vi "Open Serial Session.vi"(7 "Mode (RTU)":enum16{"RTU", "ASCII"}(ring), 8 "Error in":errorcluster caption="Error in (no error)", 9 "Slave ID":u8=1, 10 "Serial Config":T1={"baud rate (bps)"=19200, "stop bits"=10, "parity"=0, "flow control"=0, "timeout"=1000, "retries"=1} {"stop bits" items=["1.0"=10, "1.5"=15, "2.0"=20]; "flow control" items=["None", "XON/XOFF", "RTS/CTS", "XON/XOFF & RTS/CTS", "DTR/DSR", "XON/XOFF & DTR/DSR"]; "parity" items=["None", "Odd", "Even", "Mark", "Space"]}, 11 "VISA Resource":refnum<visa-resource-name>) -> (0 "Error out":errorcluster, 3 "MB_Serial session":refnum<class "MB_Master_Serial.lvclass">)   [LabVIEW 2016, in "MB Master.lvlib" / "MB_Master_Serial.lvclass"]
doc: "Opens a new modbus session and initializes the serial port. Note that the slave ID can be changed later via the property node \"Slave ID\"."
uses:
  MB_Master_Serial.lvclass
  MB_Master_Serial.lvclass/MB_Master_Serial.ctl
  MB_ADU/MB_ADU.lvclass/MB_ADU.ctl
  MB_ADU_RTU/MB_ADU_RTU.lvclass/MB_ADU_RTU.ctl
  MB_ADU/Build ADU.vi
  MB_ADU_RTU/MB_ADU_RTU.lvclass
  C:/Users/PRANAV/Downloads/Modbus-Master-master (7)/Modbus-Master-master/MB_ADU/MB_ADU.lvclass
  C:/Users/PRANAV/Downloads/Modbus-Master-master (7)/Modbus-Master-master/MB_ADU_Serial/MB_ADU_Serial.lvclass
  MB_VISA_Lock/MB_VISA_Lock.lvlib
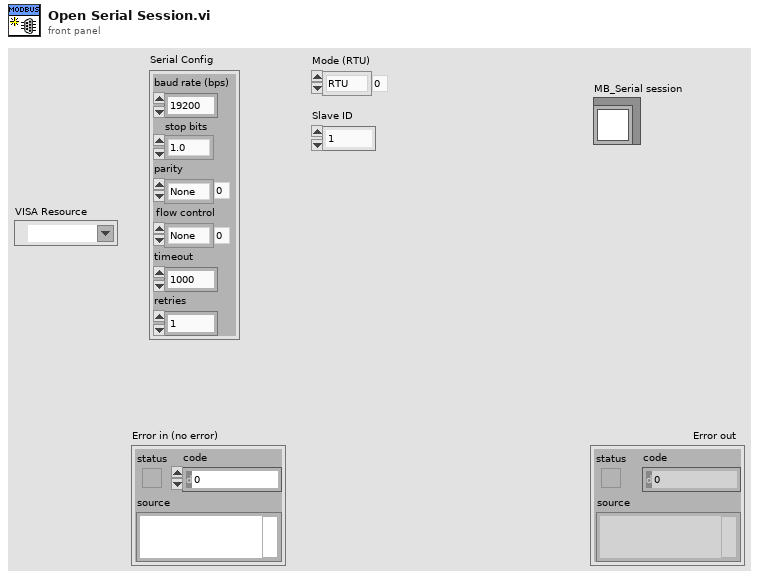
[diagram p1: front panel]
types:
  T1 = cluster{"baud rate (bps)":u32, "stop bits":u16, "parity":u16, "flow control":u16, "timeout":u32, "retries":i32}
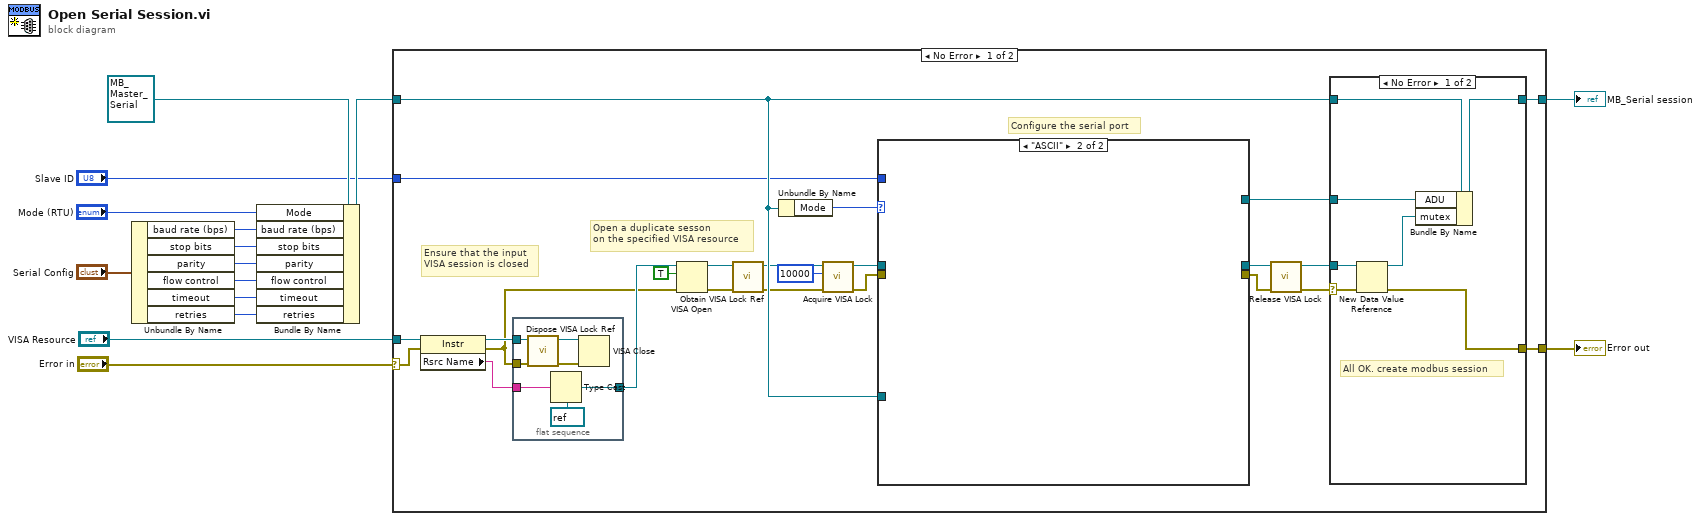
[diagram p0: block diagram]
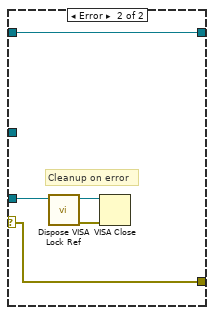
[diagram p2: hidden frame]
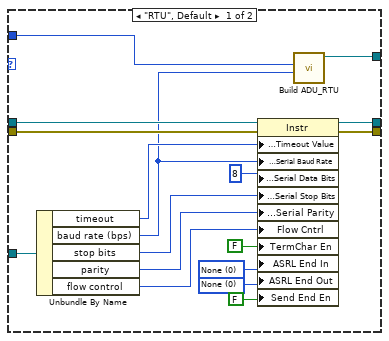
[diagram p3: hidden frame]
diagram:
  n1 = Unbundle By Name("Serial Config") -> ("baud rate (bps)"=w13:u32, "stop bits"=w12:u16, "parity"=w11:u16, "flow control"=w10:u16, "timeout"=w9:u32, "retries"=w8:i32)
  n2 = Bundle By Name(cluster=refnum<class "MB_Master_Serial.lvclass"> refnum ("MB_Serial session"), "Mode"="Mode (RTU)", "baud rate (bps)"=w13, "stop bits"=w12, "parity"=w11, "flow control"=w10, "timeout"=w9, "retries"=w8) -> (w6:refnum<class "MB_Master_Serial.lvclass">)
  n3 = case shown="No Error" "Error in" {
    selector: "Error in" -> [w31 w76]
    tunnel: [w39 w77] -> w5
    tunnel: w6 -> [w37 w77]
    tunnel: [w33 w76] -> w4
    tunnel: "Slave ID" -> [w34 _]
    tunnel: "VISA Resource" -> [w32 _]
    frame No Error {
      # "Configure the serial port"
      # "Open a duplicate sesson\non the specified VISA resource"
      # "Ensure that the input \nVISA session is closed"
      n4 = property class="Instr"(reference=w32, error in=w31) -> (reference out=w21:refnum<visa-resource-name>, error out=w18:errorcluster, "Rsrc Name"=w20:string)
      n5 = flat-sequence {
        tunnel: w21 -> [w57]
        tunnel: w18 -> [w56]
        tunnel: w20 -> [w53]
        tunnel: [w52] -> w19
        frame #0 {
          n6 = call "Dispose VISA Lock Ref.vi"("error in (no error)"=w56, "VISA session in"=w57) -> ("error out"=w55:errorcluster, "VISA session out"=w58:refnum<visa-resource-name>)  [unwired: 8 in]
          n7 = Type Cast(type=refnum<visa-resource-name> refnum ("VISA Resource"), x=w53) -> (*(type *) &x=w52:refnum<visa-resource-name>)
          n8 = VISA Close(VISA resource name=w58, error in (no error)=w55) -> ()  [unwired: 1 out]
        }
      }
      n9 = VISA Open(duplicate session (F)=TRUE, error in (no error)=w18, VISA resource name=w19) -> (VISA resource name=w30:refnum<visa-resource-name>, error out=w29:errorcluster)  [unwired: 2 in]
      n10 = call "Obtain VISA Lock Ref.vi"("error in (no error)"=w29, "VISA session in"=w30) -> ("error out"=w28:errorcluster, "VISA session out"=w27:refnum<visa-resource-name>)  [unwired: 8 in]
      n11 = Unbundle By Name(w37) -> ("Mode"=w36:enum16{"RTU", "ASCII"})
      n12 = call "Acquire VISA Lock.vi"("error in (no error)"=w28, "timeout in ms (-1)"=10000, "VISA resource name"=w27) -> ("error out"=w24:errorcluster, "VISA resource name out"=w26:refnum<visa-resource-name>)  [unwired: 7 in]
      n13 = case shown="\"ASCII\"" w36 {
        tunnel: [w61 _] -> w38
        tunnel: w26 -> [w75 _]
        tunnel: w24 -> [w74 _]
        tunnel: w37 -> [w73 _]
        tunnel: [w68 _] -> w23
        tunnel: [w63 _] -> w22
        tunnel: w34 -> [w59 _]
        frame "RTU", Default {
          w64 = u16 0 items=["None", "Last Bit", "TermChar", "Break"] ("Serial Settings:End Mode for Writes")
          w65 = u16 0 items=["None", "Last Bit", "TermChar"] ("Serial Settings:End Mode for Reads")
          n14 = Unbundle By Name(w73) -> ("timeout"=w72:u32, "baud rate (bps)"=w60:u32, "stop bits"=w71:u16, "parity"=w70:u16, "flow control"=w69:u16)
          n15 = property class="Instr"(reference=w75, error in=w74, "General Settings:Timeout Value"=w72, "Serial Settings:Serial Baud Rate"=w60, "Serial Settings:Serial Data Bits"=u16 8 ("Serial Settings:Data Bits"), "Serial Settings:Serial Stop Bits"=w71, "Serial Settings:Serial Parity"=w70, "Flow Cntrl"=w69, "TermChar En"=FALSE ("Message Based Settings:Termination Character Enable"), "ASRL End In"=w65, "ASRL End Out"=w64, "Send End En"=FALSE ("Message Based Settings:Send End Enable")) -> (reference out=w68:refnum<visa-resource-name>, error out=w63:errorcluster)
          n16 = call "Build ADU_RTU.vi"("Baud Rate (bps)"=w60, "Slave Address"=w59) -> ("MB_ADU_RTU out"=w61:refnum<class "MB_ADU_RTU.lvclass">)  [unwired: 8 in, 1 out]
        }
        frame "ASCII" {
        }
      }
      n17 = call "Release VISA Lock.vi"("error in (no error)"=w22, "VISA resource name"=w23) -> ("error out"=w16:errorcluster, "VISA resource name out"=w17:refnum<visa-resource-name>)  [unwired: 8 in]
      n18 = case shown="No Error" w16 {
        selector: w16 -> [w40 w49]
        tunnel: [w46 w48] -> w39
        tunnel: w38 -> [w45 _]
        tunnel: w37 -> [w44 w48]
        tunnel: [w43 w49] -> w33
        tunnel: w17 -> [w42 w50]
        frame No Error {
          # "All OK. create modbus session"
          n19 = New Data Value Reference(data value=w42, error in=w40) -> (data value reference=w41:refnum<data-value>, error out=w43:errorcluster)
          n20 = Bundle By Name(cluster=w44, "ADU"=w45, "mutex"=w41) -> (w46:refnum<class "MB_Master_Serial.lvclass">)
        }
        frame Error {
          # "Cleanup on error"
          n21 = call "Dispose VISA Lock Ref.vi"("VISA session in"=w50) -> ("error out"=w47:errorcluster, "VISA session out"=w51:refnum<visa-resource-name>)  [unwired: 9 in]
          n22 = VISA Close(VISA resource name=w51, error in (no error)=w47) -> ()  [unwired: 1 out]
        }
      }
    }
    frame Error {
    }
  }
  "MB_Serial session" <- w5
  "Error out" <- w4
